vi "Mysql data reader Scalar I64.vi"(8 "error in (no error)":errorcluster, 11 ".NET Refnum in":refnum<k24>) -> (0 "error out":errorcluster, 3 "GetString":i64)   [LabVIEW 2020, in "mysql.lvlib" / "mysql.lvclass"]
uses:
  mysql.lvclass
  MySql.Data
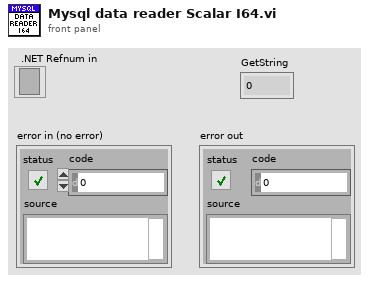
[diagram p1: front panel]
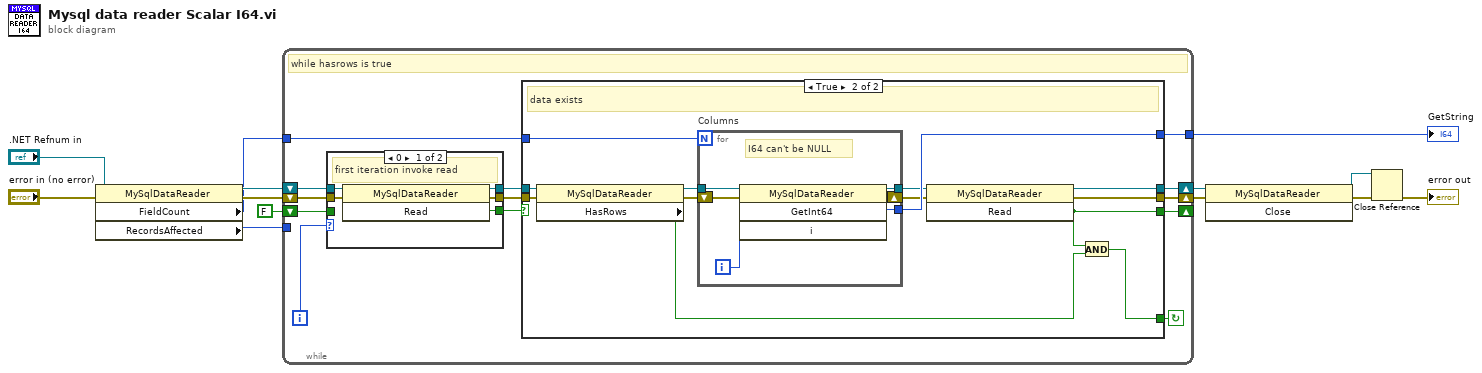
[diagram p0: block diagram]
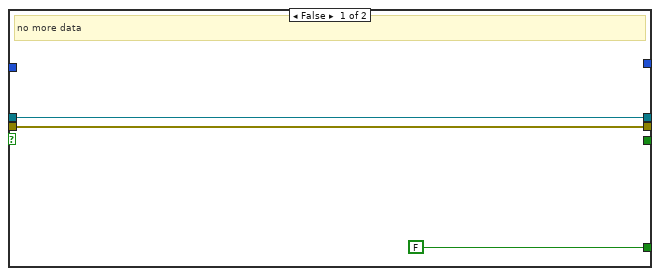
[diagram p3: hidden frame]
diagram:
  n1 = property class="MySqlDataReader"(reference=".NET Refnum in", error in="error in (no error)") -> (reference out=w8:refnum<k24>, error out=w7:errorcluster, "FieldCount"=w4:i32, "RecordsAffected"=w13:i32)
  n2 = while {
    tunnel: w4 -> [w26]
    tunnel: [w25] -> w5
    shift-right: [w23] -> w10
    shift-left: w7 -> [w21]
    shift-right: [w24] -> w9
    shift-left: w8 -> [w20]
    tunnel: w13 -> [_]
    shift-right: [w14] -> _
    shift-left: FALSE -> [w19]
    i -> [w18]
    stop <- w22 continue-if-true
    # "while hasrows is true"
    n3 = case shown="0" w18 {
      tunnel: w21 -> [w31 w33]
      tunnel: [w30 w33] -> w16
      tunnel: w20 -> [w29 w34]
      tunnel: [w28 w34] -> w15
      tunnel: [w27 w32] -> w17
      tunnel: w19 -> [_ w32]
      frame 0 {
        # "first iteration invoke read"
        n4 = invoke class="MySqlDataReader" method="Read"(reference=w29, error in=w31) -> (reference out=w28:refnum<k24>, error out=w30:errorcluster, "Read"=w27:bool)  [unwired: 1 in]
      }
      frame 1.., Default {
        # "read after for other iterations"
      }
    }
    n5 = case shown="True" w17 {
      tunnel: w26 -> [_ w50]
      tunnel: [_ w49] -> w25
      tunnel: w16 -> [w36 w48]
      tunnel: w15 -> [w37 w47]
      tunnel: [w37 w41] -> w24
      tunnel: [w36 w42] -> w23
      tunnel: [FALSE ("HasRows") w38] -> w22
      tunnel: [_ w40] -> w14
      frame False {
        # "no more data"
      }
      frame True {
        # "data exists"
        n6 = property class="MySqlDataReader"(reference=w47, error in=w48) -> (reference out=w46:refnum<k24>, error out=w45:errorcluster, "HasRows"=w39:bool)
        n7 = for "Columns" {
          N: w50 -> [_]
          tunnel: w46 -> [w51]
          shift-right: [w56] -> w44
          shift-left: w45 -> [w52]
          tunnel: [w55] -> w49
          tunnel: [w54] -> w43
          i -> [w53]
          # "I64 can't be NULL"
          n8 = invoke class="MySqlDataReader" method="GetInt64"(reference=w51, error in=w52, "i"=w53) -> (reference out=w54:refnum<k24>, error out=w56:errorcluster, "GetInt64"=w55:i64)  [unwired: 1 in, 1 out]
        }
        n9 = invoke class="MySqlDataReader" method="Read"(reference=w43, error in=w44) -> (reference out=w41:refnum<k24>, error out=w42:errorcluster, "Read"=w40:bool)  [unwired: 1 in]
        n10 = And(x=w40, y=w39) -> (x .and. y?=w38:bool)
      }
    }
  }
  "GetString" <- w5
  n11 = invoke class="MySqlDataReader" method="Close"(reference=w9, error in=w10) -> (reference out=w12:refnum<k24>, error out=w11:errorcluster)  [unwired: 1 in, 1 out]
  n12 = Close Reference(reference=w12, error in (no error)=w11) -> (error out=→"error out":errorcluster)
